vi "OBIS VISA.vi"(8 "error in (no error)":errorcluster, 10 "write to laser":string, 11 "VISA resource name":refnum<visa-resource-name>) -> (0 "error out":errorcluster, 2 "read from laser":string, 3 "VISA resource name out":refnum<visa-resource-name>)   [LabVIEW 2019, in "Coherent.lvlib"]
uses:
  Coherent.lvlib
panel:
  # "This VI sends and receives commands to the laser.  This VI is used as the lower-level communication VI for the rest of the VIs included here."
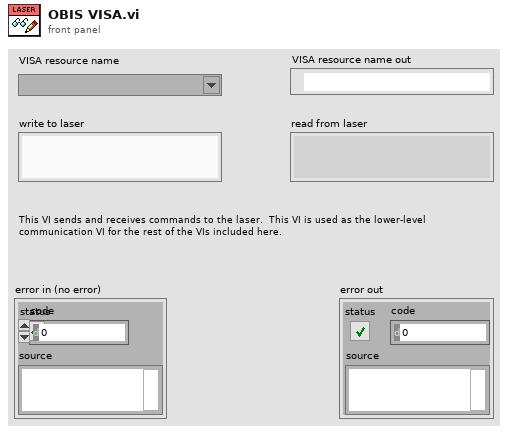
[diagram p1: front panel]
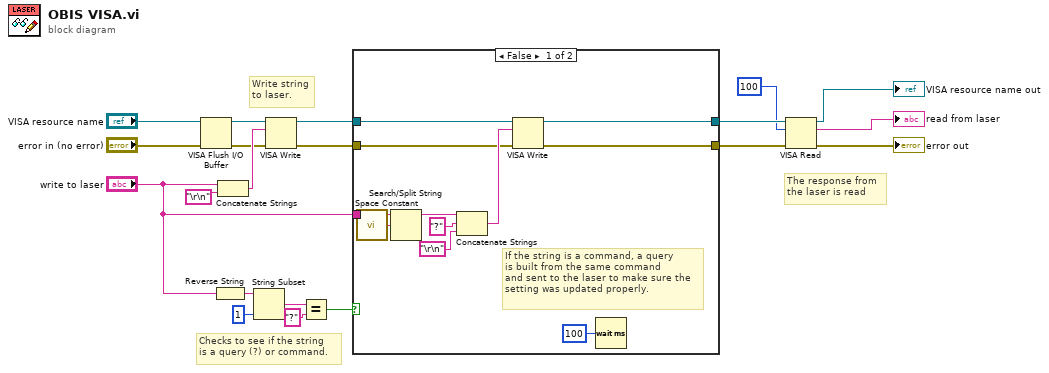
[diagram p0: block diagram]
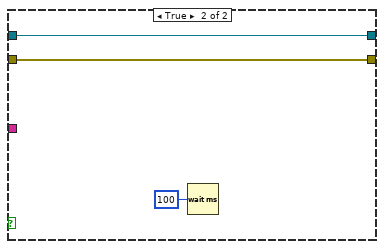
[diagram p2: hidden frame]
diagram:
  # "The response from\nthe laser is read"
  # "Checks to see if the string\nis a query (?) or command."
  # "Write string\nto laser."
  n1 = VISA Flush I/O Buffer(VISA resource name="VISA resource name", error in (no error)="error in (no error)") -> (VISA resource name out=w10:refnum<visa-resource-name>, error out=w5:errorcluster)  [unwired: 1 in]
  n2 = Reverse String(1:"write to laser") -> (0:w17:string)
  n3 = Concatenate Strings("write to laser", "\r\n") -> (w19:string)
  n4 = String Subset(string=w17, length (rest)=1 ("length (rest)")) -> (substring=w15:string)  [unwired: 1 in]
  n5 = VISA Write(VISA resource name=w10, write buffer=w19, error in (no error)=w5) -> (VISA resource name out=w18:refnum<visa-resource-name>, error out=w3:errorcluster)  [unwired: 1 out]
  n6 = Equal?(x=w15, y="?") -> (x = y?=w13:bool)
  n7 = case shown="False" w13 {
    tunnel: w18 -> [w27 w34]
    tunnel: [w26 w34] -> w12
    tunnel: "write to laser" -> [w23 _]
    tunnel: w3 -> [w22 w32]
    tunnel: [w21 w32] -> w2
    frame False {
      # "If the string is a command, a query\nis built from the same command\nand sent to the laser to make sure the\nsetting was updated properly."
      n8 = call <vilib>:"Space Constant.vi"() -> ("String"=w31:string)
      n9 = Search/Split String(string=w23, search string/char (-)=w31) -> (substring before match=w30:string)  [unwired: 1 in, 2 out]
      n10 = Concatenate Strings(w30, "?" ("string"), "\r\n") -> (w28:string)
      n11 = VISA Write(VISA resource name=w27, write buffer=w28, error in (no error)=w22) -> (VISA resource name out=w26:refnum<visa-resource-name>, error out=w21:errorcluster)  [unwired: 1 out]
      n12 = Wait (ms)(milliseconds to wait=u32 100) -> ()  [unwired: 1 out]
    }
    frame True {
      n13 = Wait (ms)(milliseconds to wait=u32 100) -> ()  [unwired: 1 out]
    }
  }
  n14 = VISA Read(VISA resource name=w12, byte count=u32 100, error in (no error)=w2) -> (VISA resource name out=→"VISA resource name out":refnum<visa-resource-name>, read buffer=→"read from laser":string, error out=→"error out":errorcluster)  [unwired: 1 out]
